vi "create do type def.vi"() -> ()   [LabVIEW 2019]
uses:
  FPGA/TypeDef/DO index.ctl
panel:
  in  "Ring":T1 items=["DO 0 [KP1 [DO 0]]", "DO 1 [ON KP2 [DO 1]]", "DO 2 [ON KP3 [DO 2]]", "DO 3 [WATER Y18.1 [DO3]]", "DO 4 [WATER Y18.2 [DO4]]", "DO 5 [KP6 Y29.1 33.7]", "DO 6 [KP7 Y29.2 33.8]", "DO 7 [KP8 Y29.3 33.9]", "DO 8 [KP9 Y29.4  33.12]", "DO 9 [KP10 Y29.5 33.1]", "DO 10 [KP11 Y29.6 33.2]", "DO 11 [KP12 Y29.7  33.13]", "DO 12 [KP13 Y29.8  33.11]", "DO 13 [KP14 Y29.9 33.10]", "DO 14 [KP15 Y29.10  33.6]", "DO 15 [KP16 Y29.11  33.5]", "DO 16 [KP17 Y29.12  33.4]", "DO 17 [KP18 Y29.13 33.3]", "DO 18 [AIR KP19]", "DO 19 [STEP DRIVE EN KP20]", "DO 20 [KP21 Y44.1 OPEN]", "DO 21 [ KP22 Y44.1 CLOSE]", "DO 22 [ KP23 Y44.2 OPEN]", "DO 23", "DO 24 [STEP DRIVE 1]", "DO 25 [STEP DRIVE 2]"]
  out "Array":string[](array[string])
  in  "DO 23":bool caption="KP24 Y44.2 抢市."
  in  "DO 22":bool caption="KP23 Y44.2 ОТК."
  in  "DO 21":bool caption="KP22 Y44.1 抢市."
  in  "DO 20":bool caption="KP21 Y44.1 ОТК."
  in  "DO 19":bool caption="Драйверы KP20"
  in  "DO 17":bool caption="KP18 Y29.13 33.3"
  in  "DO 18":bool caption="Подача воздук KP19"
  in  "DO 16":bool caption="KP17 Y29.12  33.4"
  in  "DO 15":bool caption="KP16 Y29.11  33.5"
  in  "DO 14":bool caption="KP15 Y29.10  33.6"
  in  "DO 13":bool caption="KP14 Y29.9 33.10"
  in  "DO 12":bool caption="KP13 Y29.8  33.11"
  in  "DO 11":bool caption="KP12 Y29.7  33.13"
  in  "DO 10":bool caption="KP11 Y29.6 33.2"
  in  "DO 9":bool caption="KP10 Y29.5 33.1"
  in  "DO 8":bool caption="KP9 Y29.4  33.12"
  in  "DO 7":bool caption="KP8 Y29.3 33.9"
  in  "DO 6":bool caption="KP7 Y29.2 33.8"
  in  "DO 5":bool caption="KP6 Y29.1 33.7"
  in  "DO 4":bool caption="Вода\nY18.2 [DO4]"
  in  "DO 3":bool caption="Вода\nY18.1 [DO3]"
  in  "DO 2":bool caption="Пуск\nKP3 [DO 2]"
  in  "DO 1":bool caption="Пуск\nKP2 [DO 1]"
  in  "DO 0":bool caption="KP1 [DO 0]"
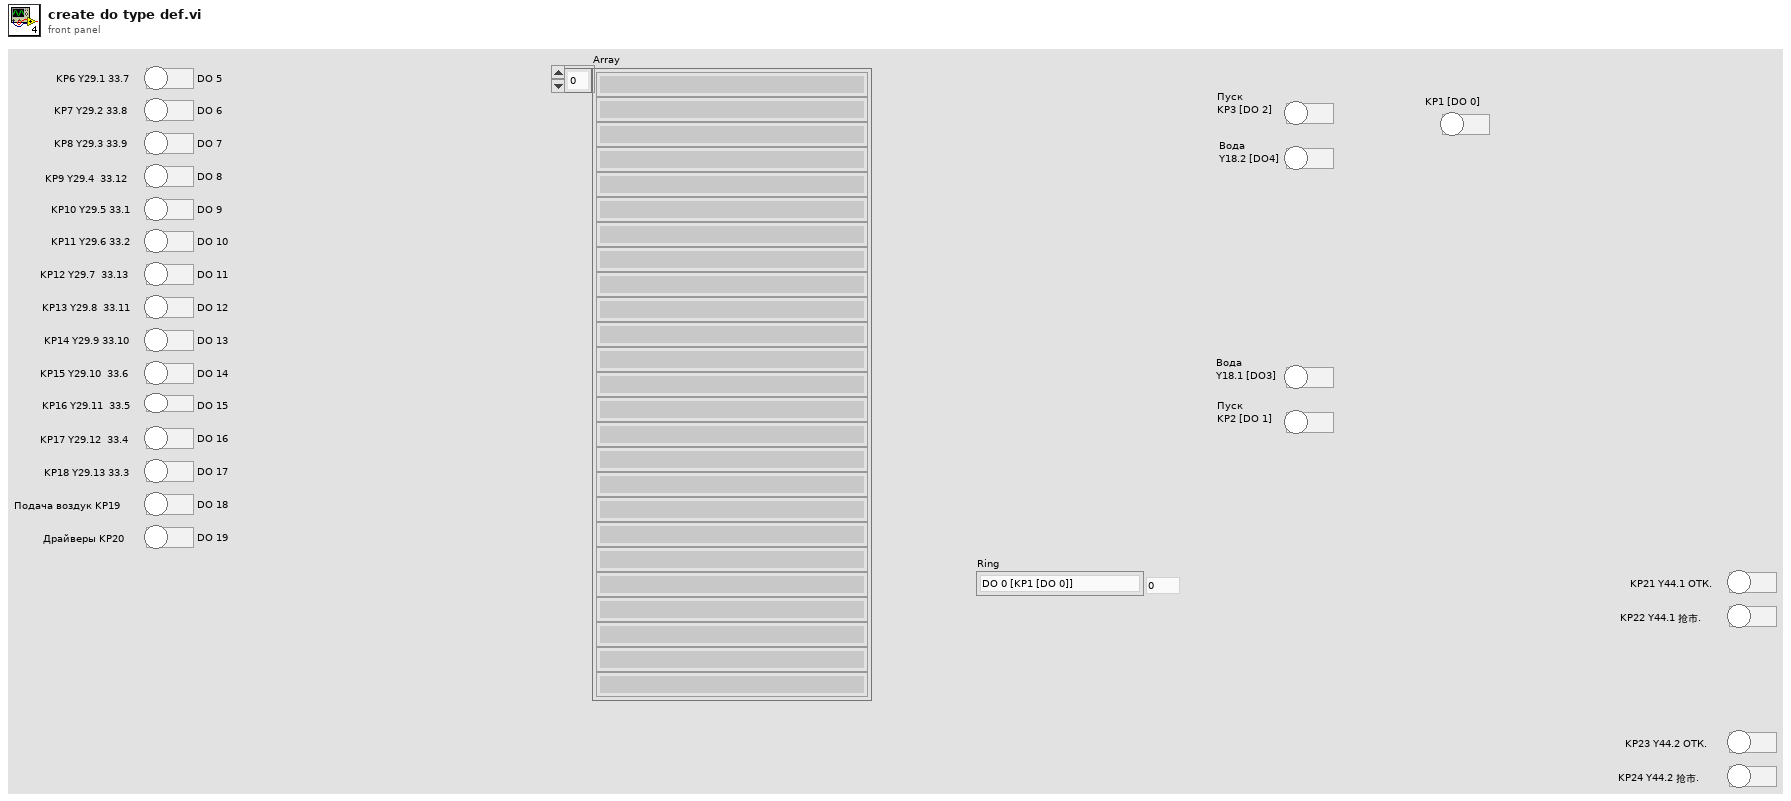
[diagram p1: front panel]
types:
  T1 = typedef "DO index.ctl" = u8
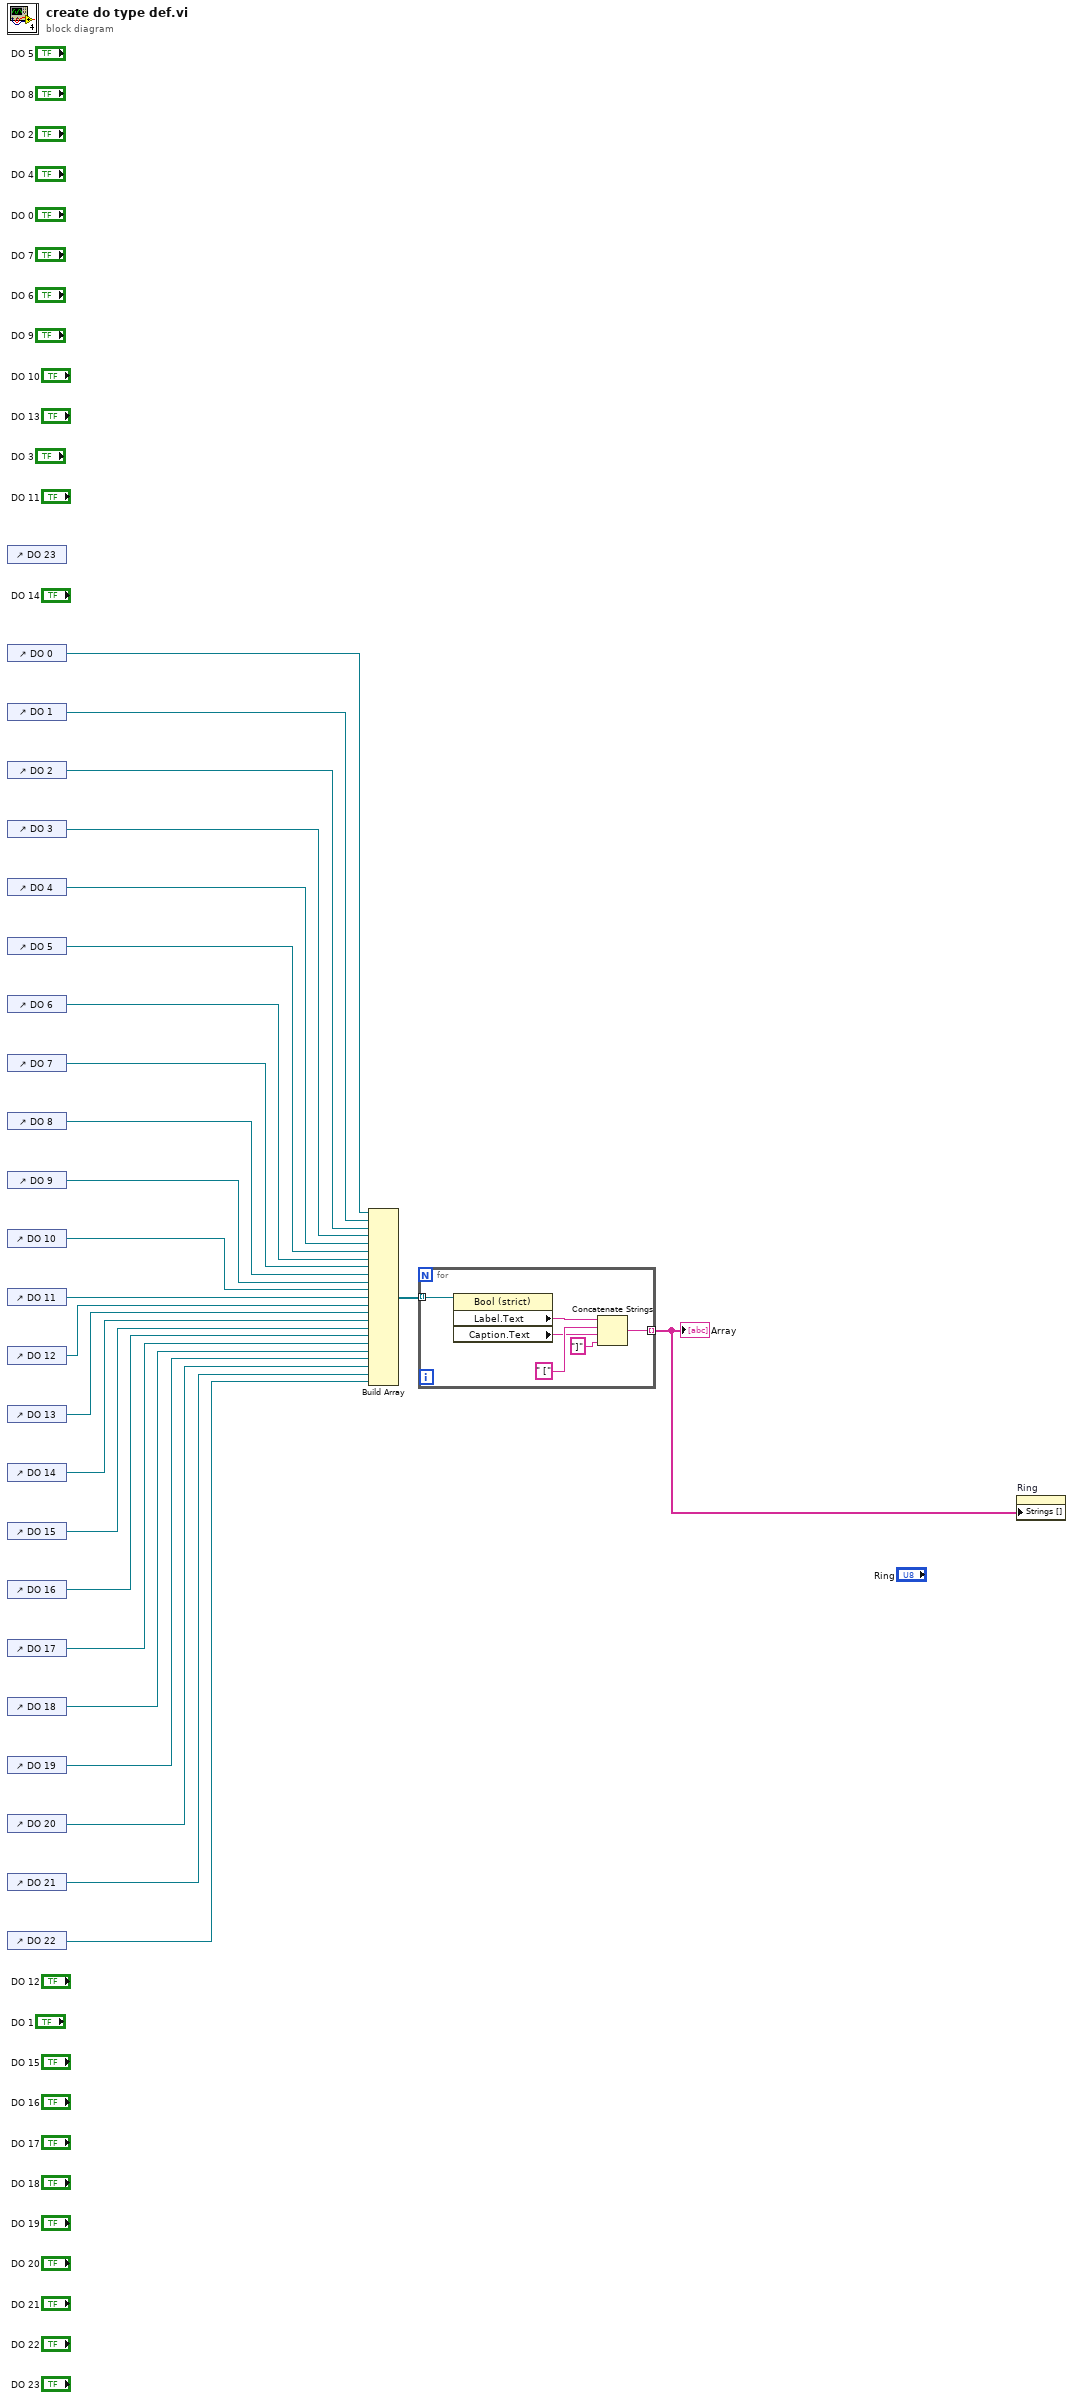
[diagram p0: block diagram]
diagram:
  n1 = control-ref of="DO 23"() -> ()  [unwired: 1 out]
  n2 = control-ref of="DO 0"() -> (w25:refnum<vi>)
  n3 = control-ref of="DO 1"() -> (w24:refnum<vi>)
  n4 = control-ref of="DO 2"() -> (w23:refnum<vi>)
  n5 = control-ref of="DO 3"() -> (w22:refnum<vi>)
  n6 = control-ref of="DO 4"() -> (w21:refnum<vi>)
  n7 = control-ref of="DO 5"() -> (w20:refnum<vi>)
  n8 = control-ref of="DO 6"() -> (w19:refnum<vi>)
  n9 = control-ref of="DO 7"() -> (w18:refnum<vi>)
  n10 = control-ref of="DO 8"() -> (w17:refnum<vi>)
  n11 = control-ref of="DO 9"() -> (w16:refnum<vi>)
  n12 = control-ref of="DO 10"() -> (w15:refnum<vi>)
  n13 = control-ref of="DO 11"() -> (w14:refnum<vi>)
  n14 = control-ref of="DO 12"() -> (w13:refnum<vi>)
  n15 = control-ref of="DO 13"() -> (w12:refnum<vi>)
  n16 = control-ref of="DO 14"() -> (w11:refnum<vi>)
  n17 = control-ref of="DO 15"() -> (w10:refnum<vi>)
  n18 = control-ref of="DO 16"() -> (w9:refnum<vi>)
  n19 = control-ref of="DO 17"() -> (w8:refnum<vi>)
  n20 = control-ref of="DO 18"() -> (w7:refnum<vi>)
  n21 = control-ref of="DO 19"() -> (w6:refnum<vi>)
  n22 = control-ref of="DO 20"() -> (w5:refnum<vi>)
  n23 = control-ref of="DO 21"() -> (w4:refnum<vi>)
  n24 = control-ref of="DO 22"() -> (w3:refnum<vi>)
  n25 = Build Array(w25, w24, w23, w22, w21, w20, w19, w18, w17, w16, w15, w14, w13, w12, w11, w10, w9, w8, w7, w6, w5, w4, w3) -> (w2:refnum<vi>[])
  n26 = for {
    tunnel: w2 -> [w31] mode=indexing
    tunnel: [w27] -> w1 mode=indexing
    n27 = property class="Bool (strict)"(reference=w31) -> ("Label.Text"=w30:string, "Caption.Text"=w28:string)  [unwired: 1 in, 2 out]
    n28 = Concatenate Strings(w30, " [" ("string"), w28, "]" ("string")) -> (w27:string)
  }
  "Array" <- w1
  n29 = property on="Ring" class="Ring (strict)"("Strings []"=w1) -> ()  [unwired: 2 in, 2 out]
